vi "2. FGV Write and read.vi"(8 "error in (no error)":errorcluster, 9 "Timeout (s)":dbl, 10 "Command":string="H", 11 "VISA resource name":refnum<visa-resource-name>="COM3") -> (0 "error out":errorcluster)   [LabVIEW 2014]
uses:
  control/FGV Serial Tasks.ctl
panel:
  out "que hay":u8
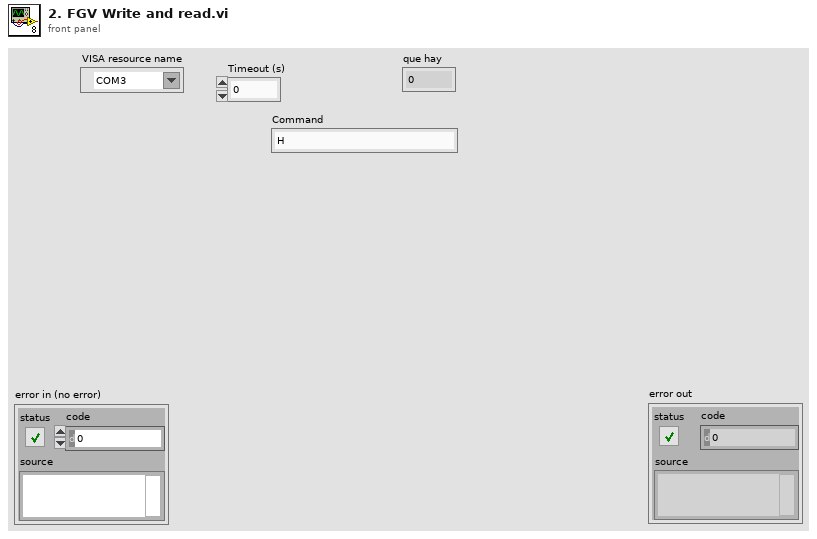
[diagram p1: front panel]
types:
  T1 = typedef "FGV Serial Tasks.ctl" = enum16{"Open", "Read", "Write", "Close", "Flush"}
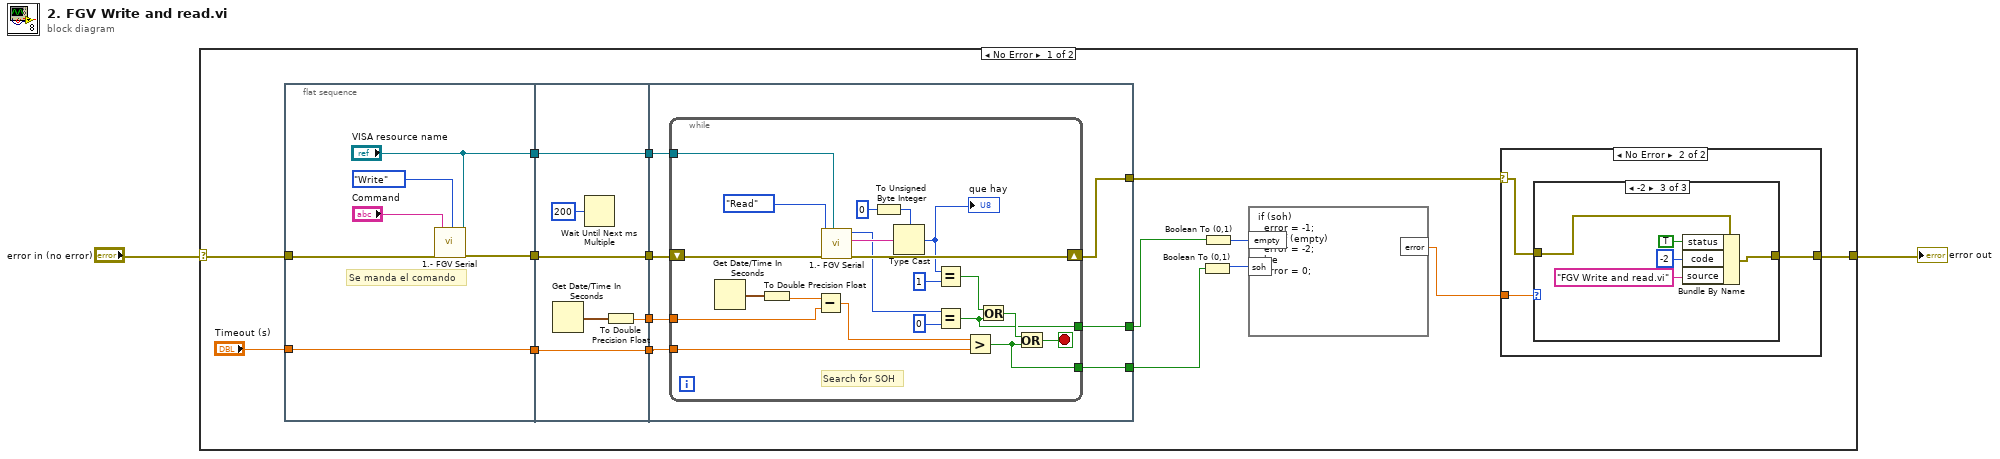
[diagram p0: block diagram]
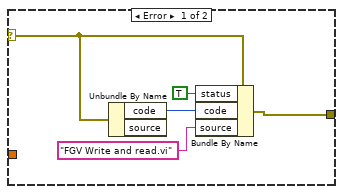
[diagram p2: hidden frame]
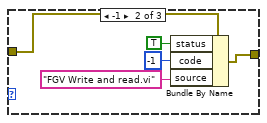
[diagram p4: hidden frame]
diagram:
  n1 = case shown="No Error" "error in (no error)" {
    selector: "error in (no error)" -> [w17 w78]
    tunnel: [w18 w78] -> w1
    frame No Error {
      n2 = flat-sequence {
        tunnel: [w42] -> w16
        tunnel: w17 -> [w43]
        tunnel: ["VISA resource name"] -> w13
        tunnel: [w39] -> w9
        tunnel: "Timeout (s)" -> [w39]
        tunnel: w16 -> [w48]
        tunnel: [w48] -> w15
        tunnel: [w47] -> w14
        tunnel: w13 -> [w47]
        tunnel: [w45] -> w11
        tunnel: [w44] -> w10
        tunnel: w9 -> [w44]
        tunnel: w15 -> [w55]
        tunnel: w14 -> [w56]
        tunnel: [w54] -> w12
        tunnel: w11 -> [w53]
        tunnel: w10 -> [w52]
        tunnel: [w51] -> w5
        tunnel: [w50] -> w4
        frame #0 {
          # "Se manda el comando"
          n3 = call "1.- FGV Serial.vi"("VISA resource name"="VISA resource name", "error in (no error)"=w43, "Command"="Command", "Task"=FGV_Serial_Tasks."Write") -> ("error out"=w42:errorcluster)  [unwired: 5 in, 2 out]
        }
        frame #1 {
          n4 = Get Date/Time In Seconds() -> (seconds since 1Jan1904=w46:timestamp)
          n5 = Wait Until Next ms Multiple(millisecond multiple=u32 200) -> ()  [unwired: 1 out]
          n6 = To Double Precision Float(number=w46) -> (double precision float=w45:dbl)
        }
        frame #2 {
          n7 = while {
            tunnel: w56 -> [w76]
            shift-right: [w74] -> w54
            shift-left: w55 -> [w75]
            tunnel: w53 -> [w65]
            tunnel: w52 -> [w63]
            tunnel: [w58] -> w51
            tunnel: [w57] -> w50
            stop <- w68 stop-if-true
            # "Search for SOH"
            n8 = Get Date/Time In Seconds() -> (seconds since 1Jan1904=w67:timestamp)
            n9 = To Double Precision Float(number=w67) -> (double precision float=w66:dbl)
            n10 = Subtract(x=w66, y=w65) -> (x-y=w64:dbl)
            n11 = call "1.- FGV Serial.vi"("VISA resource name"=w76, "error in (no error)"=w75, "Task"=FGV_Serial_Tasks."Read") -> ("error out"=w74:errorcluster, "Receive buffer"=w73:string, "return count"=w61:u32)  [unwired: 6 in]
            n12 = To Unsigned Byte Integer(number=u8 0) -> (unsigned 8bit integer=w72:u8)
            n13 = Type Cast(type=w72, x=w73) -> (*(type *) &x=w70:u8)
            "que hay" <- w70
            n14 = Equal?(x=w70, y=u8 1) -> (x = y?=w60:bool)
            n15 = Equal?(x=w61, y=u8 0) -> (x = y?=w57:bool)
            n16 = Greater?(x=w64, y=w63) -> (0:w58:bool)
            n17 = Or(x=w60, y=w57) -> (x .or. y?=w59:bool)
            n18 = Or(x=w59, y=w58) -> (x .or. y?=w68:bool)
          }
        }
      }
      n19 = Boolean To (0,1)(Boolean=w5) -> (0, 1=w6:i16)
      n20 = Boolean To (0,1)(Boolean=w4) -> (0, 1=w7:i16)
      n21 = formula code="if (soh)\n  error = -1;\nelse if (empty)\n  error = -2;\nelse\n  error = 0;"("soh"=w6, "empty"=w7) -> ("error"=w3:dbl)
      n22 = case shown="No Error" w12 {
        selector: w12 -> [w22 w25]
        tunnel: [w21 w24] -> w18
        tunnel: w3 -> [_ w26]
        frame Error {
          n23 = Unbundle By Name(w22) -> ("code"=w23:i32)  [unwired: 1 out]
          n24 = Bundle By Name(cluster=w22, "status"=TRUE, "code"=w23, "source"="FGV Write and read.vi") -> (w21:errorcluster)
        }
        frame No Error {
          n25 = case shown="-2" w26 {
            tunnel: [w27 w28 w34] -> w24
            tunnel: w25 -> [w27 w29 w33]
            frame 0, Default {
            }
            frame -1 {
              n26 = Bundle By Name(cluster=w29, "status"=TRUE, "code"=-1, "source"="FGV Write and read.vi") -> (w28:errorcluster)
            }
            frame -2 {
              n27 = Bundle By Name(cluster=w33, "status"=TRUE, "code"=-2, "source"="FGV Write and read.vi") -> (w34:errorcluster)
            }
          }
        }
      }
    }
    frame Error {
    }
  }
  "error out" <- w1
